vi "Set LOG flag.vi"(8 "error in (no error)":errorcluster, 11 "ICS in":refnum<class "ICS.lvclass">) -> (0 "error out":errorcluster, 3 "ICS out":refnum<class "ICS.lvclass">)   [LabVIEW 2018, in "ICS.lvclass"]
uses:
  ICS.lvclass
  ICS.lvclass/ICS.ctl
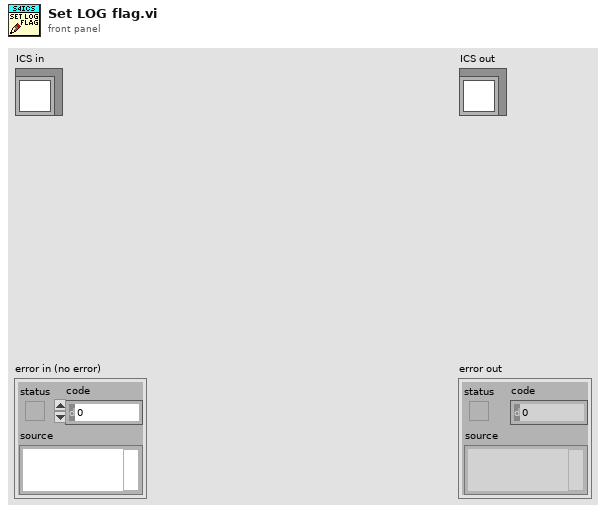
[diagram p1: front panel]
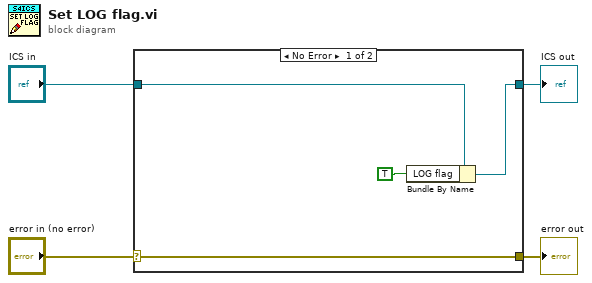
[diagram p0: block diagram]
diagram:
  n1 = case shown="No Error" "error in (no error)" {
    selector: "error in (no error)" -> [w8 w9]
    tunnel: [w8 w9] -> w3
    tunnel: [w6 w10] -> w1
    tunnel: "ICS in" -> [w7 w10]
    frame No Error {
      n2 = Bundle By Name(cluster=w7, "LOG flag"=TRUE) -> (w6:refnum<class "ICS.lvclass">)
    }
    frame Error {
    }
  }
  "error out" <- w3
  "ICS out" <- w1
